vi "CCD_Exposure.vi"(0 "CCD Parameters":T2={"Exposure Time (s)"=0.2, "Offset"=0.0, "BkgrdCrct"=FALSE, "Shutter"=FALSE, "Mode"=enum."Regular", "Repetition"=4, "dt or s"=0.0} {"dt or s" format="%#.6f"; "Repetition" min=1; "Offset" format="%#.2f"; "Exposure Time (s)" min=0.02 max=6000.0 format="%#.2f"}, 11 "error in":errorcluster) -> (4 "PixelOverflow":bool, 6 "#PixelOverflow":u32, 8 "Array Length":i32=1024, 10 "The Data":dbl[](array[numeric])=[1198.0, 1190.0, 1193.0, 1194.0, 1189.0, 1188.0, 1196.0, 1190.0, 1202.0, 1191.0, 1193.0, 1192.0, 1199.0, 1189.0, 1194.0, 1189.0, 1197.0, 1191.0, 1187.0, 1192.0, 1195.0, 1189.0, 1195.0, 1191.0, 1199.0, 1194.0, 1192.0, 1191.0, 1193.0, 1197.0, 1193.0, 1193.0, 1194.0, 1200.0, 1191.0, 1190.0, 1187.0, 1195.0, 1189.0, 1188.0, 1191.0, 1194.0, 1187.0, 1192.0, 1198.0, 1193.0, 1190.0, 1192.0, 1190.0, 1193.0, 1191.0, 1190.0, 1191.0, 1189.0, 1192.0, 1194.0, 1190.0, 1193.0, 1193.0, 1191.0, 1194.0, 1182.0, 1190.0, 1188.0, 1199.0, 1192.0, 1196.0, 1195.0, 1186.0, 1189.0, 1188.0, 1185.0, 1194.0, 1187.0, 1193.0, 1194.0, 1190.0, 1189.0, 1189.0, 1187.0, 1196.0, 1195.0, 1191.0, 1197.0, 1192.0, 1200.0, 1187.0, 1194.0, 1189.0, 1193.0, 1195.0, 1196.0, 1186.0, 1192.0, 1190.0, 1194.0, 1194.0, 1190.0, 1191.0, 1193.0, 1197.0, 1197.0, 1185.0, 1199.0, 1190.0, 1195.0, 1196.0, 1184.0, 1193.0, 1193.0, 1193.0, 1191.0, 1189.0, 1190.0, 1199.0, 1193.0, 1191.0, 1194.0, 1191.0, 1192.0, 1186.0, 1190.0, 1194.0, 1189.0, 1194.0, 1190.0, 1191.0, 1192.0, 1192.0, 1196.0, 1192.0, 1192.0, 1189.0, 1193.0, 1198.0, 1186.0, 1191.0, 1193.0, 1187.0, 1194.0, 1190.0, 1190.0, 1191.0, 1189.0, 1194.0, 1195.0, 1189.0, 1192.0, 1185.0, 1193.0, 1192.0, 1192.0, 1189.0, 1191.0, 1191.0, 1190.0, 1196.0, 1194.0, 1193.0, 1191.0, 1189.0, 1191.0, 1196.0, 1192.0, 1192.0, 1189.0, 1196.0, 1191.0, 1193.0, 1192.0, 1188.0, 1190.0, 1194.0, 1192.0, 1185.0, 1191.0, 1194.0, 1191.0, 1189.0, 1195.0, 1192.0, 1196.0, 1190.0, 1193.0, 1191.0, 1189.0, 1194.0, 1195.0, 1191.0, 1187.0, 1190.0, 1196.0, 1196.0, 1192.0, 1197.0, 1191.0, 1189.0, 1192.0, 1192.0, 1200.0, 1192.0, 1193.0, 1190.0, 1192.0, 1187.0, 1198.0, 1186.0, 1196.0, 1201.0, 1199.0, 1200.0, 1191.0, 1196.0, 1200.0, 1192.0, 1191.0, 1193.0, 1185.0, 1192.0, 1194.0, 1186.0, 1190.0, 1188.0, 1189.0, 1201.0, 1197.0, 1191.0, 1194.0, 1193.0, 1194.0, 1195.0, 1198.0, 1200.0, 1192.0, 1192.0, 1193.0, 1193.0, 1195.0, 1187.0, 1193.0, 1192.0, 1187.0, 1189.0, 1186.0, 1191.0, 1197.0, 1191.0, 1200.0, 1194.0, 1192.0, 1187.0, 1196.0, 1191.0, 1191.0, 1196.0, 1187.0, 1190.0, 1193.0, 1189.0, 1193.0, 1190.0, 1188.0, 1188.0, 1190.0, 1197.0, 1188.0, 1191.0, 1195.0, 1188.0, 1191.0, 1188.0, 1194.0, 1193.0, 1187.0, 1200.0, 1192.0, 1197.0, 1190.0, 1196.0, 1200.0, 1191.0, 1189.0, 1193.0, 1189.0, 1186.0, 1196.0, 1185.0, 1198.0, 1195.0, 1186.0, 1191.0, 1197.0, 1191.0, 1193.0, 1195.0, 1193.0, 1191.0, 1198.0, 1189.0, 1183.0, 1200.0, 1197.0, 1192.0, 1192.0, 1192.0, 1196.0, 1191.0, 1190.0, 1194.0, 1188.0, 1198.0, 1193.0, 1195.0, 1190.0, 1187.0, 1192.0, 1191.0, 1195.0, 1188.0, 1190.0, 1191.0, 1187.0, 1189.0, 1185.0, 1189.0, 1196.0, 1198.0, 1191.0, 1190.0, 1196.0, 1197.0, 1193.0, 1187.0, 1186.0, 1195.0, 1191.0, 1193.0, 1192.0, 1196.0, 1190.0, 1192.0, 1192.0, 1192.0, 1190.0, 1195.0, 1192.0, 1191.0, 1193.0, 1197.0, 1184.0, 1190.0, 1188.0, 1192.0, 1194.0, 1190.0, 1193.0, 1195.0, 1195.0, 1194.0, 1189.0, 1193.0, 1191.0, 1194.0, 1186.0, 1189.0, 1192.0, 1191.0, 1182.0, 1190.0, 1197.0, 1194.0, 1188.0, 1193.0, 1191.0, 1186.0, 1194.0, 1197.0, 1193.0, 1191.0, 1187.0, 1194.0, 1194.0, 1191.0, 1189.0, 1195.0, 1194.0, 1189.0, 1196.0, 1187.0, 1186.0, 1192.0, 1194.0, 1196.0, 1191.0, 1193.0, 1191.0, 1188.0, 1190.0, 1199.0, 1198.0, 1196.0, 1196.0, 1190.0, 1194.0, 1191.0, 1194.0, 1187.0, 1195.0, 1190.0, 1194.0, 1196.0, 1194.0, 1189.0, 1193.0, 1189.0, 1194.0, 1189.0, 1195.0, 1192.0, 1194.0, 1193.0, 1191.0, 1197.0, 1187.0, 1189.0, 1189.0, 1188.0, 1197.0, 1192.0, 1189.0, 1193.0, 1194.0, 1183.0, 1202.0, 1187.0, 1192.0, 1184.0, 1188.0, 1186.0, 1193.0, 1189.0, 1195.0, 1189.0, 1193.0, 1197.0, 1189.0, 1194.0, 1191.0, 1194.0, 1192.0, 1191.0, 1191.0, 1196.0, 1194.0, 1190.0, 1193.0, 1192.0, 1195.0, 1197.0, 1198.0, 1193.0, 1202.0, 1196.0, 1194.0, 1194.0, 1190.0, 1193.0, 1190.0, 1195.0, 1192.0, 1187.0, 1194.0, 1197.0, 1190.0, 1194.0, 1189.0, 1198.0, 1192.0, 1191.0, 1192.0, 1192.0, 1191.0, 1191.0, 1193.0, 1191.0, 1191.0, 1198.0, 1186.0, 1192.0, 1185.0, 1185.0, 1188.0, 1194.0, 1196.0, 1194.0, 1195.0, 1190.0, 1194.0, 1191.0, 1190.0, 1195.0, 1191.0, 1191.0, 1195.0, 1192.0, 1194.0, 1201.0, 1187.0, 1191.0, 1195.0, 1187.0, 1192.0, 1192.0, 1193.0, 1200.0, 1188.0, 1189.0, 1189.0, 1197.0, 1189.0, 1188.0, 1197.0, 1195.0, 1191.0, 1189.0, 1190.0, 1195.0, 1189.0, 1191.0, 1194.0, 1186.0, 1192.0, 1190.0, 1191.0, 1188.0, 1195.0, 1192.0, 1191.0, 1191.0, 1199.0, 1190.0, 1190.0, 1190.0, 1192.0, 1187.0, 1193.0, 1197.0, 1197.0, 1186.0, 1193.0, 1189.0, 1192.0, 1197.0, 1184.0, 1187.0, 1188.0, 1192.0, 1192.0, 1192.0, 1189.0, 1192.0, 1190.0, 1194.0, 1191.0, 1186.0, 1196.0, 1194.0, 1189.0, 1193.0, 1191.0, 1186.0, 1189.0, 1193.0, 1195.0, 1196.0, 1197.0, 1199.0, 1194.0, 1190.0, 1193.0, 1194.0, 1190.0, 1198.0, 1196.0, 1194.0, 1195.0, 1194.0, 1184.0, 1188.0, 1195.0, 1197.0, 1190.0, 1194.0, 1190.0, 1191.0, 1195.0, 1198.0, 1188.0, 1193.0, 1194.0, 1195.0, 1198.0, 1195.0, 1191.0, 1197.0, 1192.0, 1198.0, 1190.0, 1196.0, 1191.0, 1194.0, 1188.0, 1189.0, 1198.0, 1192.0, 1198.0, 1195.0, 1185.0, 1191.0, 1193.0, 1192.0, 1197.0, 1195.0, 1195.0, 1195.0, 1193.0, 1190.0, 1190.0, 1190.0, 1198.0, 1195.0, 1191.0, 1194.0, 1190.0, 1190.0, 1194.0, 1194.0, 1195.0, 1192.0, 1190.0, 1194.0, 1195.0, 1192.0, 1192.0, 1194.0, 1189.0, 1192.0, 1193.0, 1188.0, 1194.0, 1195.0, 1196.0, 1193.0, 1192.0, 1201.0, 1191.0, 1198.0, 1197.0, 1191.0, 1192.0, 1191.0, 1194.0, 1193.0, 1188.0, 1192.0, 1189.0, 1183.0, 1189.0, 1190.0, 1192.0, 1189.0, 1196.0, 1193.0, 1197.0, 1185.0, 1193.0, 1189.0, 1191.0, 1196.0, 1195.0, 1193.0, 1193.0, 1191.0, 1189.0, 1193.0, 1192.0, 1192.0, 1192.0, 1190.0, 1191.0, 1193.0, 1193.0, 1197.0, 1195.0, 1189.0, 1193.0, 1188.0, 1194.0, 1197.0, 1194.0, 1195.0, 1196.0, 1190.0, 1194.0, 1188.0, 1197.0, 1195.0, 1191.0, 1195.0, 1192.0, 1194.0, 1188.0, 1190.0, 1197.0, 1197.0, 1191.0, 1187.0, 1197.0, 1191.0, 1193.0, 1188.0, 1191.0, 1194.0, 1193.0, 1195.0, 1192.0, 1195.0, 1189.0, 1193.0, 1193.0, 1195.0, 1190.0, 1192.0, 1196.0, 1188.0, 1187.0, 1193.0, 1192.0, 1192.0, 1194.0, 1185.0, 1199.0, 1190.0, 1193.0, 1191.0, 1198.0, 1189.0, 1190.0, 1191.0, 1190.0, 1193.0, 1195.0, 1186.0, 1190.0, 1193.0, 1191.0, 1189.0, 1197.0, 1193.0, 1198.0, 1190.0, 1192.0, 1193.0, 1191.0, 1196.0, 1193.0, 1196.0, 1190.0, 1190.0, 1198.0, 1192.0, 1199.0, 1198.0, 1190.0, 1191.0, 1191.0, 1196.0, 1190.0, 1196.0, 1195.0, 1191.0, 1196.0, 1195.0, 1193.0, 1190.0, 1190.0, 1195.0, 1193.0, 1187.0, 1197.0, 1185.0, 1191.0, 1189.0, 1191.0, 1193.0, 1192.0, 1188.0, 1196.0, 1193.0, 1191.0, 1193.0, 1193.0, 1190.0, 1192.0, 1192.0, 1192.0, 1195.0, 1191.0, 1195.0, 1189.0, 1189.0, 1191.0, 1191.0, 1185.0, 1192.0, 1191.0, 1193.0, 1201.0, 1199.0, 1197.0, 1206.0, 1201.0, 1207.0, 1200.0, 1198.0, 1195.0, 1188.0, 1194.0, 1186.0, 1190.0, 1197.0, 1188.0, 1193.0, 1196.0, 1193.0, 1192.0, 1192.0, 1188.0, 1196.0, 1186.0, 1193.0, 1194.0, 1188.0, 1190.0, 1190.0, 1192.0, 1190.0, 1191.0, 1191.0, 1200.0, 1192.0, 1199.0, 1193.0, 1190.0, 1190.0, 1199.0, 1187.0, 1193.0, 1190.0, 1188.0, 1194.0, 1194.0, 1196.0, 1194.0, 1195.0, 1190.0, 1187.0, 1187.0, 1196.0, 1193.0, 1199.0, 1190.0, 1193.0, 1193.0, 1191.0, 1198.0, 1192.0, 1193.0, 1192.0, 1193.0, 1189.0, 1189.0, 1197.0, 1189.0, 1194.0, 1193.0, 1192.0, 1185.0, 1198.0, 1193.0, 1189.0, 1192.0, 1193.0, 1196.0, 1190.0, 1195.0, 1189.0, 1196.0, 1198.0, 1190.0, 1191.0, 1193.0, 1186.0, 1189.0, 1195.0, 1188.0, 1197.0, 1188.0, 1191.0, 1185.0, 1190.0, 1193.0, 1188.0, 1198.0, 1192.0, 1193.0, 1194.0, 1194.0, 1189.0, 1184.0, 1193.0, 1199.0, 1193.0, 1192.0, 1193.0, 1190.0, 1196.0, 1191.0, 1192.0, 1189.0, 1194.0, 1188.0, 1189.0, 1190.0, 1190.0, 1192.0, 1195.0, 1188.0, 1190.0, 1192.0, 1189.0, 1197.0, 1192.0, 1194.0, 1187.0, 1196.0, 1192.0, 1194.0, 1185.0, 1187.0, 1187.0, 1191.0, 1195.0, 1190.0, 1186.0, 1183.0, 1194.0, 1194.0, 1192.0, 1192.0, 1188.0, 1193.0, 1195.0, 1189.0, 1190.0, 1191.0, 1192.0, 1196.0, 1186.0, 1195.0, 1191.0, 1185.0, 1191.0, 1187.0, 1190.0, 1188.0, 1189.0, 1187.0, 1196.0, 1191.0, 1190.0, 1191.0, 1190.0, 1196.0, 1195.0, 1186.0, 1187.0, 1187.0, 1188.0, 1194.0, 1192.0, 1192.0, 1192.0, 1189.0, 1192.0, 1191.0, 1188.0, 1188.0, 1187.0, 1187.0, 1190.0, 1186.0, 1191.0, 1195.0, 1192.0, 1196.0, 1193.0, 1192.0, 1191.0, 1189.0, 1187.0, 1193.0, 1188.0, 1189.0, 1194.0, 1191.0, 1185.0, 1193.0, 1191.0, 1196.0, 1196.0, 1199.0, 1195.0, 1211.0] format="%.2f", 14 "GPIB Status":i16=-1, 15 "Error Out":errorcluster)   [LabVIEW 2021]
doc: "This is the controlling VI for CCD exposures.\nIt calls the right CCD subVIs if the \"Current Experiment Status\" Exposure status is \"OK\".\nIt will also set the \"Current Experiment Status\" Exposure status \nfrom \"OK\" to \"Busy\" to \"Done\" ."
uses:
  Globals and TypeDefs/Type Definitions.llb/CCDParameter.ctt
  Globals and TypeDefs/Type Definitions.llb/ListOfDetectors.ctt
  Globals and TypeDefs/Type Definitions.llb/3 way Status.ctl
  Globals and TypeDefs/gStatus.vi
panel:
  in  "Current Detector":T1
  out "Plot":dbl[](graph)
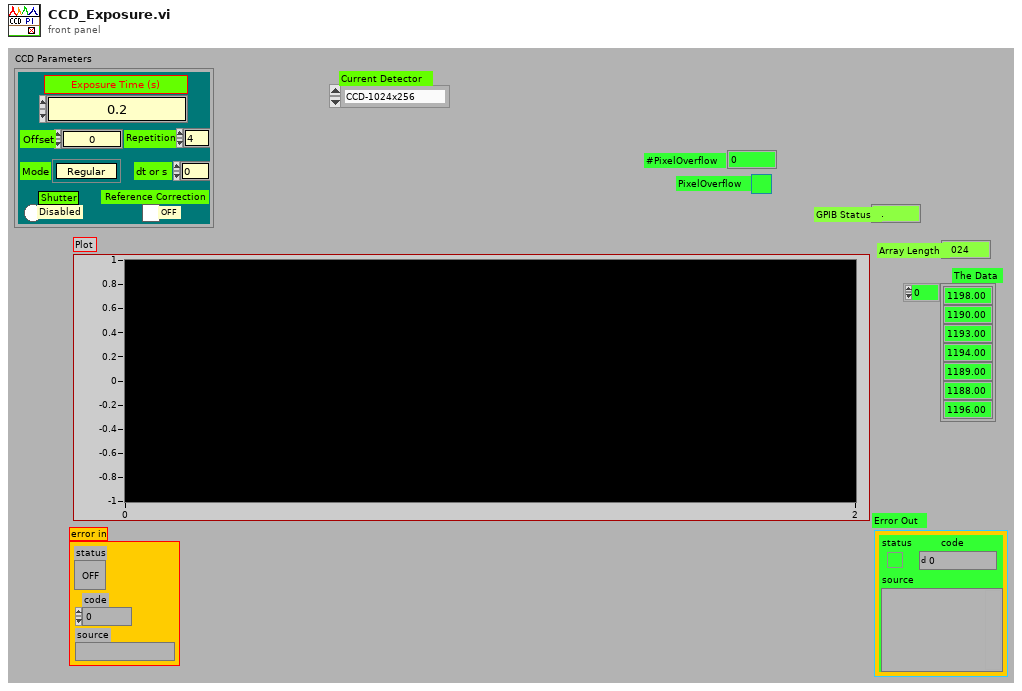
[diagram p1: front panel]
types:
  T1 = typedef "ListOfDetectors.ctt" = enum8{"CCD-1024x256", "InGaAs PDA-1024x1", "CCD-1340x400", "Ge Single Channel", "Si Single Channel", "PMT Single Channel"}
  T2 = typedef "CCDParameter.ctt" = cluster{"Exposure Time (s)":dbl, "Offset":dbl, "BkgrdCrct":bool, "Shutter":bool, "Mode":enum8{"Regular", "OverExp Cor", "SpikeRemove", "ForCalibration"}, "Repetition":u16, "dt or s":dbl}
  T3 = enum8{"Regular", "OverExp Cor", "SpikeRemove", "ForCalibration"}
  T4 = typedef "3 way Status.ctl" = u8
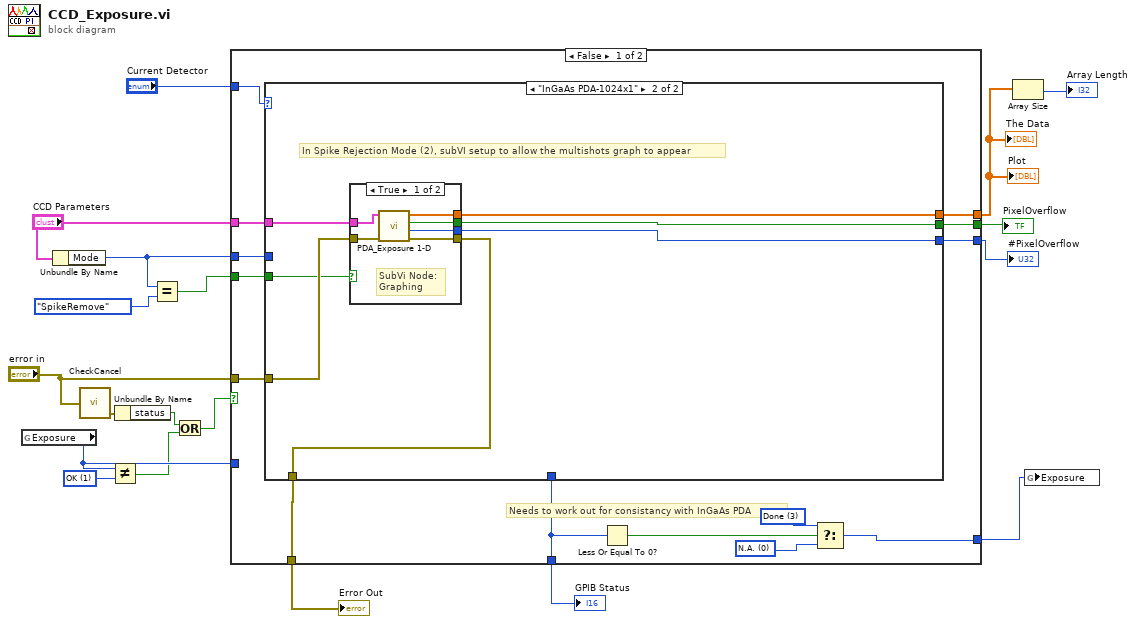
[diagram p0: block diagram]
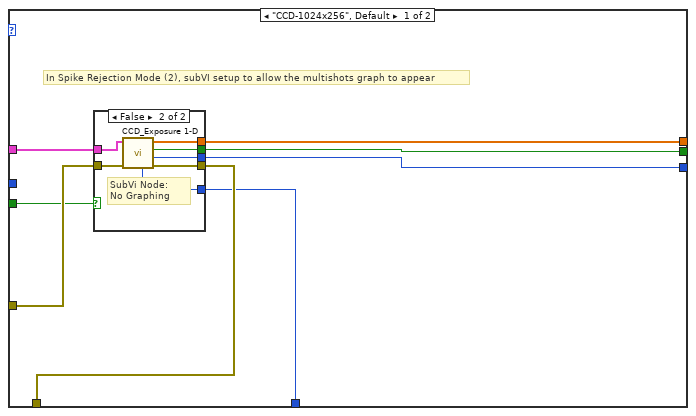
[diagram p2: hidden frame]
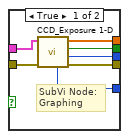
[diagram p3: hidden frame]
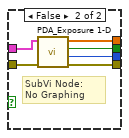
[diagram p4: hidden frame]
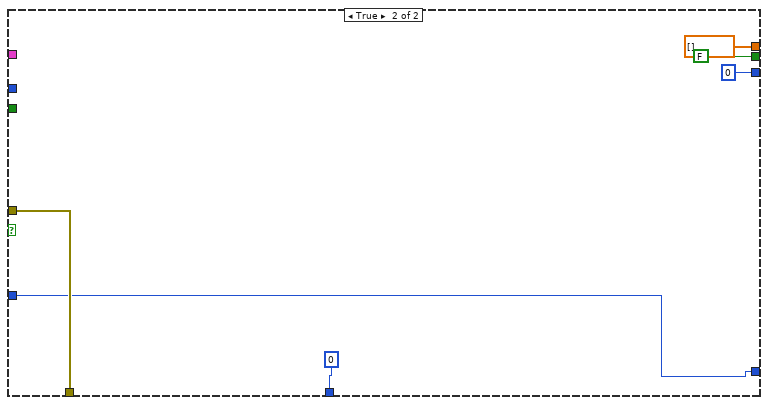
[diagram p5: hidden frame]
diagram:
  w13 = T4 1 items=["N.A.", "OK", "Busy", "Done"] ("Exposure")
  n1 = global read "gStatus.vi" "Exposure"() -> (w6:T4)
  n2 = Unbundle By Name("CCD Parameters") -> ("Mode"=w11:T3)
  n3 = call "CheckCancel.vi"("error in (no error)"="error in") -> ("error out"=w5:errorcluster)  [unwired: 1 in, 1 out]
  n4 = Not Equal?(x=w6, y=w13) -> (x != y?=w3:bool)
  n5 = Unbundle By Name(w5) -> ("status"=w4:bool)
  n6 = Equal?(x=w11, y=T3."SpikeRemove") -> (x = y?=w12:bool)
  n7 = Or(x=w4, y=w3) -> (x .or. y?=w2:bool)
  n8 = case shown="False" w2 {
    tunnel: [w30 w80] -> w19
    tunnel: "error in" -> [w31 w80]
    tunnel: "Current Detector" -> [w33 _]
    tunnel: w11 -> [w32 _]
    tunnel: [w29 dbl[] [] ("The Data")] -> w15
    tunnel: [w28 FALSE ("PixelOverflow")] -> w18
    tunnel: [w27 u32 0 ("#PixelOverflow")] -> w17
    tunnel: [w23 i16 0 ("GPIB Status")] -> w16
    tunnel: w6 -> [_ w75]
    tunnel: w12 -> [w24 _]
    tunnel: [w21 w75] -> w1
    tunnel: "CCD Parameters" -> [w20 _]
    frame False {
      w25 = T4 0 items=["N.A.", "OK", "Busy", "Done"] ("Exposure")
      w26 = T4 3 items=["N.A.", "OK", "Busy", "Done"] ("Exposure")
      # "Needs to work out for consistancy with InGaAs PDA"
      n9 = case shown="\"InGaAs PDA-1024x1\"" w33 {
        tunnel: w32 -> [_ _]
        tunnel: w31 -> [w41 w62]
        tunnel: [w40 w61] -> w30
        tunnel: [w39 w60] -> w29
        tunnel: [w38 w59] -> w28
        tunnel: [w37 w58] -> w27
        tunnel: [w36 _] -> w23
        tunnel: w24 -> [w35 w57]
        tunnel: w20 -> [w34 w56]
        frame "CCD-1024x256", Default {
          # "In Spike Rejection Mode (2), subVI setup to allow the multishots graph to appear"
          n10 = case shown="False" w35 {
            tunnel: w41 -> [w48 w55]
            tunnel: [w47 w54] -> w40
            tunnel: [w46 w53] -> w39
            tunnel: [w45 w52] -> w38
            tunnel: [w44 w51] -> w37
            tunnel: [w43 w50] -> w36
            tunnel: w34 -> [w42 w49]
            frame True {
              # "SubVi Node:\nGraphing"
              n11 = call "CCD_Exposure 1-D.vi"("error in"=w48, "CCD Parameters"=w42) -> ("Error Out"=w47:errorcluster, "#PixelOverflow"=w44:u32, "PixelOverflow"=w45:bool, "The Data"=w46:dbl[], "GPIB Status"=w43:i16)  [unwired: 3 in, 2 out]
            }
            frame False {
              # "SubVi Node:\nNo Graphing"
              n12 = call "CCD_Exposure 1-D.vi"("error in"=w55, "CCD Parameters"=w49) -> ("Error Out"=w54:errorcluster, "#PixelOverflow"=w51:u32, "PixelOverflow"=w52:bool, "The Data"=w53:dbl[], "GPIB Status"=w50:i16)  [unwired: 3 in, 2 out]
            }
          }
        }
        frame "InGaAs PDA-1024x1" {
          # "In Spike Rejection Mode (2), subVI setup to allow the multishots graph to appear"
          n13 = case shown="True" w57 {
            tunnel: w62 -> [w68 w74]
            tunnel: [w67 w73] -> w61
            tunnel: [w66 w72] -> w60
            tunnel: [w65 w71] -> w59
            tunnel: [w64 w70] -> w58
            tunnel: w56 -> [w63 w69]
            frame True {
              # "SubVi Node:\nGraphing"
              n14 = call "PDA_Exposure 1-D.vi"("error in"=w68, "CCD Parameters"=w63) -> ("Error Out"=w67:errorcluster, "#PixelOverflow"=w64:u32, "PixelOverflow"=w65:bool, "The Data"=w66:dbl[])  [unwired: 5 in, 1 out]
            }
            frame False {
              # "SubVi Node:\nNo Graphing"
              n15 = call "PDA_Exposure 1-D.vi"("error in"=w74, "CCD Parameters"=w69) -> ("Error Out"=w73:errorcluster, "#PixelOverflow"=w70:u32, "PixelOverflow"=w71:bool, "The Data"=w72:dbl[])  [unwired: 5 in, 1 out]
            }
          }
        }
      }
      n16 = Less Or Equal To 0?(x=w23) -> (x <= 0?=w22:bool)
      n17 = Select(t=w26, s=w22, f=w25) -> (s? t:f=w21:T4)
    }
    frame True {
    }
  }
  "Error Out" <- w19
  "The Data" <- w15
  "Plot" <- w15
  "PixelOverflow" <- w18
  "#PixelOverflow" <- w17
  "GPIB Status" <- w16
  n18 = Array Size(array=w15) -> (size(s)=→"Array Length":i32)
  n19 = global write "gStatus.vi" "Exposure"(w1) -> ()
